vi "MAVLink CRC v2 Generate.vi"(11 "Message":u8[](array[numeric]) format="%x") -> (3 "Message w/ CRC":u8[](array[numeric]))   [LabVIEW 2014]
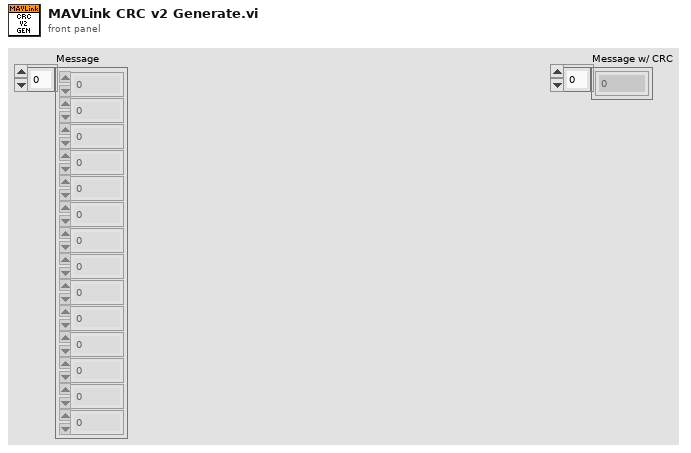
[diagram p1: front panel]
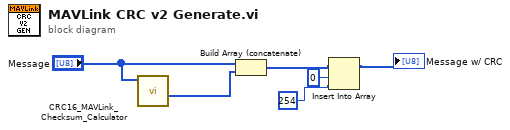
[diagram p0: block diagram]
diagram:
  n1 = call "CRC16_MAVLink_Checksum_Calculator.vi"("Message"="Message") -> ("Bytes"=w5:u8[])  [unwired: 9 in, 1 out]
  n2 = Build Array (concatenate)("Message", w5) -> (w4:u8[])
  n3 = Insert Into Array(array=w4, index=0, new element=u8 254) -> (→"Message w/ CRC":u8[])
